vi "Server Log Stuff.vi"(7 "log (true)":bool, 8 "error in":errorcluster, 9 "write/read (false:write)":bool, 10 "String":string, 11 "log ref":refnum<vi>) -> (0 "error out":errorcluster)   [LabVIEW 2013]
doc: "Add record to server log."
uses:
  <vilib>/Utility/error.llb/whitespace.ctl
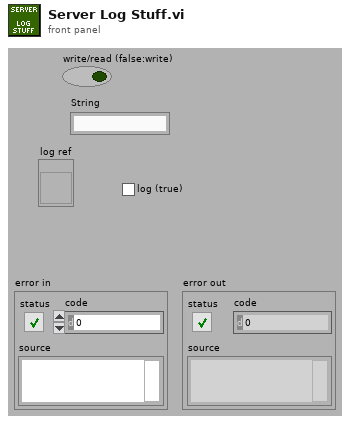
[diagram p1: front panel]
types:
  T1 = typedef "whitespace.ctl" = u16
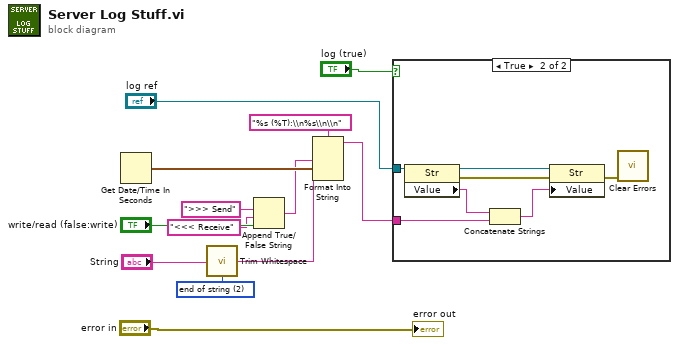
[diagram p0: block diagram]
diagram:
  w6 = T1 2 items=["both", "start of string", "end of string"] ("location (both)")
  n1 = Get Date/Time In Seconds() -> (seconds since 1Jan1904=w13:timestamp)
  n2 = call <vilib>:"Trim Whitespace.vi"("string"="String", "location (both)"=w6) -> ("trimmed string"=w5:string)
  n3 = Append True/False String(1:"write/read (false:write)", 2:"<<< Receive" ("false string"), 3:">>> Send" ("true string")) -> (0:w9:string)  [unwired: 1 in]
  n4 = Format Into String(format string="%s (%T):\\n%s\\n\\n", w9, w13, w5) -> (resulting string=w3:string)  [unwired: 2 in, 1 out]
  n5 = case shown="True" "log (true)" {
    tunnel: w3 -> [_ w17]
    tunnel: "log ref" -> [_ w15]
    frame False {
    }
    frame True {
      n6 = property class="Str"(reference=w15) -> (reference out=w19:refnum<vi>, error out=w20:errorcluster, "Value"=w18:string)  [unwired: 1 in]
      n7 = Concatenate Strings(w18, w17) -> (w16:string)
      n8 = property class="Str"(reference=w19, error in=w20, "Value"=w16) -> (error out=w14:errorcluster)  [unwired: 1 out]
      n9 = call <vilib>:"Clear Errors.vi"("error in (no error)"=w14) -> ()  [unwired: 6 in, 1 out]
    }
  }
  "error out" <- "error in"
